vi "axex_get_list_of_workbooks.vi"(8 "error in":errorcluster, 11 "names ring ref":refnum<vi>) -> (0 "error out":errorcluster, 1 "Excel not running":bool, 2 "names":string[](array[string]), 3 "full paths":string[](array[string]))   [LabVIEW 2020, in "AX Excel.lvlib"]
doc: "Returns list of opened workbooks. Will not generate error."
uses:
  AX Excel.lvlib
  axex_get_list_of_workbooks_proc.vi
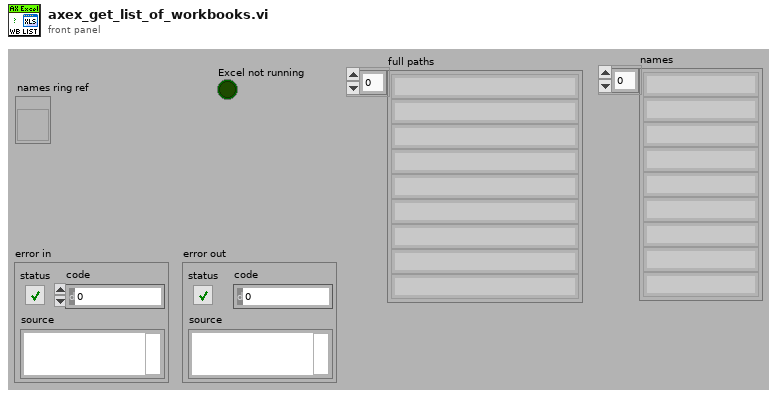
[diagram p1: front panel]
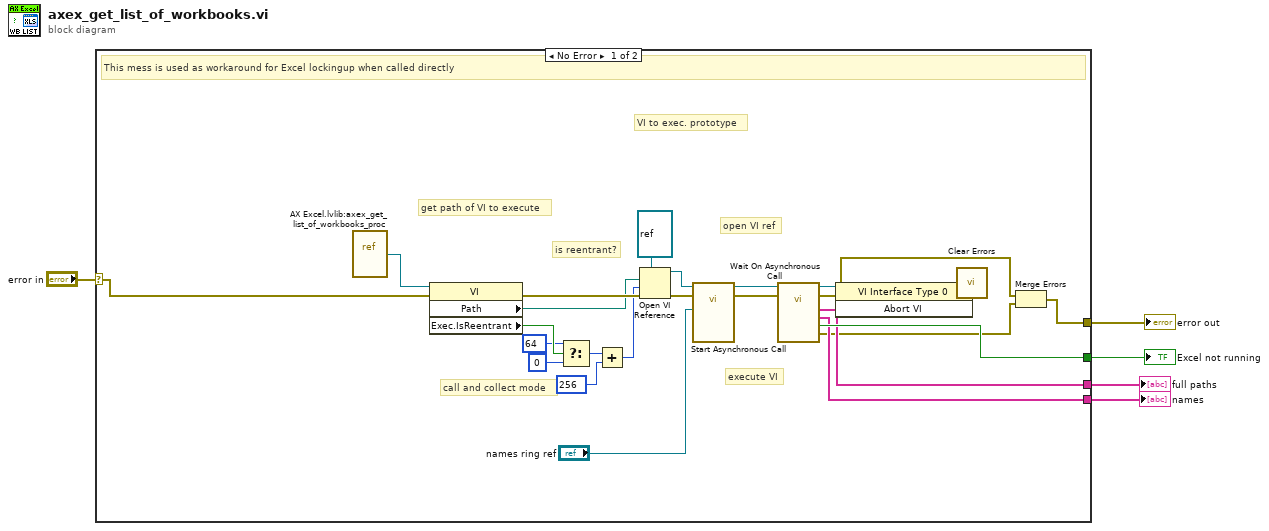
[diagram p0: block diagram]
diagram:
  n1 = case shown="No Error" "error in" {
    selector: "error in" -> [w15 w30]
    tunnel: [w11 w30] -> w5
    tunnel: [w14 _] -> w3
    tunnel: [w13 _] -> w2
    tunnel: [w12 _] -> w1
    frame No Error {
      # "execute VI"
      # "open VI ref"
      # "VI to exec. prototype"
      # "get path of VI to execute"
      # "is reentrant?"
      # "call and collect mode"
      # "This mess is used as workaround for Excel lockingup when called directly"
      n2 = vi-ref "AX Excel.lvlib:axex_get_list_of_workbooks_proc.vi"() -> (w9:refnum<vi>)
      n3 = property class="VI"(reference=w9, error in=w15) -> (error out=w29:errorcluster, "Path"=w28:path, "Exec.IsReentrant"=w24:bool)  [unwired: 1 out]
      n4 = Select(t=64 ("options"), s=w24, f=0 ("options")) -> (s? t:f=w23:i32)
      n5 = Add(x=w23, y=256 ("options")) -> (x+y=w19:i32)
      n6 = Open VI Reference(type specifier VI Refnum (for type only)=refnum<vi> refnum, vi path=w28, options=w19, error in (no error)=w29) -> (vi reference=w25:refnum<vi>, error out=w26:errorcluster)  [unwired: 2 in]
      n7 = call-by-ref "Start Asynchronous Call"(reference=w25, error in=w26, "names ring ref"="names ring ref") -> (reference out=w16:refnum<vi>, error out=w17:errorcluster)  [unwired: 7 in, 4 out]
      n8 = call-by-ref "Wait On Asynchronous Call"(reference=w16, error in=w17) -> (reference out=w8:refnum<vi>, error out=w7:errorcluster, 0:"error out"=w10:errorcluster, "Excel not running"=w14:bool, "names"=w12:string[], "full paths"=w13:string[])  [unwired: 8 in]
      n9 = invoke class="VI Interface Type 0" method="Abort VI"(reference=w8) -> (error out=w6:errorcluster)  [unwired: 2 in, 2 out]
      n10 = call <vilib>:"Clear Errors.vi"("error in (no error)"=w6) -> ()  [unwired: 5 in, 2 out]
      n11 = Merge Errors(w7, w10) -> (w11:errorcluster)
    }
    frame Error {
    }
  }
  "error out" <- w5
  "Excel not running" <- w3
  "full paths" <- w2
  "names" <- w1
